vi "Untitled 1.vi"() -> ()   [LabVIEW 2020, in "PostgreSQL Driver.lvlib"]
uses:
  PostgreSQL Driver.lvlib
  <vilib>/addons/database/Connection.llb/DB Tools Open Connec (String).vi
  <vilib>/addons/database/NI_Database_API.lvlib
panel:
  out "Query Time":dbl format="%#_6f"
  in  "error in (no error)":errorcluster
  in  "DSN":string
  in  "password":string
  in  "userID":string
  in  "SQL query":string
  out "data":string[][](array[string])
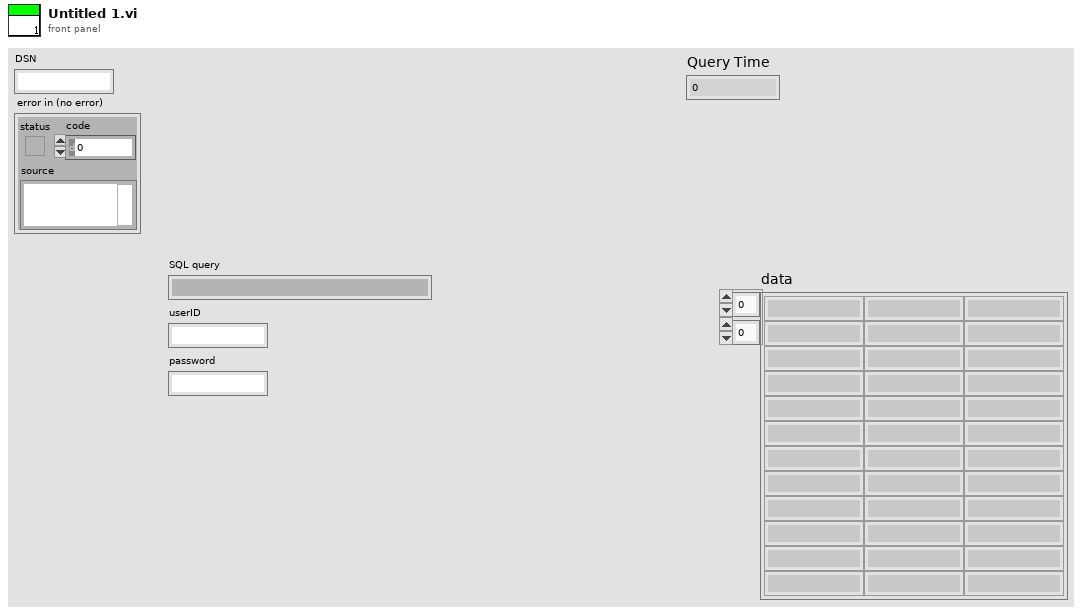
[diagram p1: front panel]
types:
  T1 = typedef "NI_Database_API.lvlib/Conn ObjectReference.ctl" = refnum<k1>
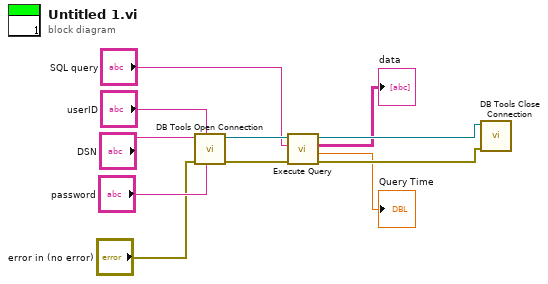
[diagram p0: block diagram]
diagram:
  n1 = call-poly <vilib>:"DB Tools Open Connection.vi"("password"="password", "userID"="userID", "error in (no error)"="error in (no error)", "connection information"="DSN") -> ("error out"=w8:errorcluster, "connection reference"=w9:T1)  [unwired: 4 in]
  n2 = call "Execute Query.vi"("error in (no error)"=w8, "SQL query"="SQL query", "Refnum in"=w9) -> ("error out"=w10:errorcluster, "Query Time"=→"Query Time":dbl, "data"=→"data":string[][], "Refnum out"=w11:T1)  [unwired: 5 in]
  n3 = call <vilib>:"DB Tools Close Connection.vi"("error in (no error)"=w10, "connection reference"=w11) -> ()  [unwired: 5 in, 1 out]
